vi "FaulhaberV3-Ascii_V1.vi"() -> (1 "searchnames":string[](array[string]), 2 "ID":u32[](array[numeric]), 3 "Faulhaber Objects":T3(array[cluster]))   [LabVIEW 2011] (continued)
"Default"="0", "Kommentart"=""}, {"ID"=621150254, "Name"="Encoder compensation_Value 45", "type"=enum."S16", "rw"=enum."rw", "lowLimit"="-32768", "highLimit"="32767", "Default"="0", "Kommentart"=""}, {"ID"=621150255, "Name"="Encoder compensation_Value 46", "type"=enum."S16", "rw"=enum."rw", "lowLimit"="-32768", "highLimit"="32767", "Default"="0", "Kommentart"=""}, {"ID"=621150256, "Name"="Encoder compensation_Value 47", "type"=enum."S16", "rw"=enum."rw", "lowLimit"="-32768", "highLimit"="32767", "Default"="0", "Kommentart"=""}, {"ID"=621150257, "Name"="Encoder compensation_Value 48", "type"=enum."S16", "rw"=enum."rw", "lowLimit"="-32768", "highLimit"="32767", "Default"="0", "Kommentart"=""}, {"ID"=621150258, "Name"="Encoder compensation_Value 49", "type"=enum."S16", "rw"=enum."rw", "lowLimit"="-32768", "highLimit"="32767", "Default"="0", "Kommentart"=""}, {"ID"=621150259, "Name"="Encoder compensation_Value 50", "type"=enum."S16", "rw"=enum."rw", "lowLimit"="-32768", "highLimit"="32767", "Default"="0", "Kommentart"=""}, {"ID"=621150260, "Name"="Encoder compensation_Value 51", "type"=enum."S16", "rw"=enum."rw", "lowLimit"="-32768", "highLimit"="32767", "Default"="0", "Kommentart"=""}, {"ID"=621150261, "Name"="Encoder compensation_Value 52", "type"=enum."S16", "rw"=enum."rw", "lowLimit"="-32768", "highLimit"="32767", "Default"="0", "Kommentart"=""}, {"ID"=621150262, "Name"="Encoder compensation_Value 53", "type"=enum."S16", "rw"=enum."rw", "lowLimit"="-32768", "highLimit"="32767", "Default"="0", "Kommentart"=""}, {"ID"=621150263, "Name"="Encoder compensation_Value 54", "type"=enum."S16", "rw"=enum."rw", "lowLimit"="-32768", "highLimit"="32767", "Default"="0", "Kommentart"=""}, {"ID"=621150264, "Name"="Encoder compensation_Value 55", "type"=enum."S16", "rw"=enum."rw", "lowLimit"="-32768", "highLimit"="32767", "Default"="0", "Kommentart"=""}, {"ID"=621150265, "Name"="Encoder compensation_Value 56", "type"=enum."S16", "rw"=enum."rw", "lowLimit"="-32768", "highLimit"="32767", "Default"="0", "Kommentart"=""}, {"ID"=621150266, "Name"="Encoder compensation_Value 57", "type"=enum."S16", "rw"=enum."rw", "lowLimit"="-32768", "highLimit"="32767", "Default"="0", "Kommentart"=""}, {"ID"=621150267, "Name"="Encoder compensation_Value 58", "type"=enum."S16", "rw"=enum."rw", "lowLimit"="-32768", "highLimit"="32767", "Default"="0", "Kommentart"=""}, {"ID"=621150268, "Name"="Encoder compensation_Value 59", "type"=enum."S16", "rw"=enum."rw", "lowLimit"="-32768", "highLimit"="32767", "Default"="0", "Kommentart"=""}, {"ID"=621150269, "Name"="Encoder compensation_Value 60", "type"=enum."S16", "rw"=enum."rw", "lowLimit"="-32768", "highLimit"="32767", "Default"="0", "Kommentart"=""}, {"ID"=621150270, "Name"="Encoder compensation_Value 61", "type"=enum."S16", "rw"=enum."rw", "lowLimit"="-32768", "highLimit"="32767", "Default"="0", "Kommentart"=""}, {"ID"=621150271, "Name"="Encoder compensation_Value 62", "type"=enum."S16", "rw"=enum."rw", "lowLimit"="-32768", "highLimit"="32767", "Default"="0", "Kommentart"=""}, {"ID"=621150272, "Name"="Encoder compensation_Value 63", "type"=enum."S16", "rw"=enum."rw", "lowLimit"="-32768", "highLimit"="32767", "Default"="0", "Kommentart"=""}, {"ID"=621412352, "Name"="Pwm frequency", "type"=enum."U8", "rw"=enum."rw", "lowLimit"="1", "highLimit"="10", "Default"="4", "Kommentart"=""}, {"ID"=621740032, "Name"="250F_00", "type"=enum."U8", "rw"=enum."wo", "lowLimit"="0", "highLimit"="255", "Default"="0", "Kommentart"=""}, {"ID"=637534208, "Name"="Drive system gear_Number of entries", "type"=enum."U8", "rw"=enum."ro", "lowLimit"="", "highLimit"="", "Default"="2", "Kommentart"=""}, {"ID"=637534209, "Name"="Drive system gear_Gear ratio num", "type"=enum."U32", "rw"=enum."rw", "lowLimit"="1", "highLimit"="4294967295", "Default"="1", "Kommentart"=""}, {"ID"=637534210, "Name"="Drive system gear_Gear ratio den", "type"=enum."U32", "rw"=enum."rw", "lowLimit"="1", "highLimit"="4294967295", "Default"="1", "Kommentart"=""}, {"ID"=637599744, "Name"="Drive system load transmission_Number of entries", "type"=enum."U8", "rw"=enum."ro", "lowLimit"="", "highLimit"="", "Default"="3", "Kommentart"=""}, {"ID"=637599745, "Name"="Drive system load transmission_Load transmission", "type"=enum."U8", "rw"=enum."rw", "lowLimit"="0", "highLimit"="255", "Default"="", "Kommentart"=""}, {"ID"=637599746, "Name"="Drive system load transmission_Load transmission ratio num", "type"=enum."U32", "rw"=enum."rw", "lowLimit"="1", "highLimit"="4294967295", "Default"="1", "Kommentart"=""}, {"ID"=637599747, "Name"="Drive system load transmission_Load transmission ratio den", "type"=enum."U32", "rw"=enum."rw", "lowLimit"="1", "highLimit"="4294967295", "Default"="1", "Kommentart"=""}, {"ID"=637665280, "Name"="Drive system numbers_Number of entries", "type"=enum."U8", "rw"=enum."ro", "lowLimit"="", "highLimit"="", "Default"="3", "Kommentart"=""}, {"ID"=637665281, "Name"="Drive system numbers_Gear catalog number", "type"=enum."string", "rw"=enum."rw", "lowLimit"="", "highLimit"="", "Default"="0", "Kommentart"=""}, {"ID"=637665282, "Name"="Drive system numbers_Encoder cataloge number", "type"=enum."string", "rw"=enum."rw", "lowLimit"="", "highLimit"="", "Default"="0", "Kommentart"=""}, {"ID"=637665283, "Name"="Drive system numbers_Drive combination number", "type"=enum."string", "rw"=enum."rw", "lowLimit"="", "highLimit"="", "Default"="0", "Kommentart"=""}, {"ID"=637730816, "Name"="Drive system units_Number of entries", "type"=enum."U8", "rw"=enum."ro", "lowLimit"="", "highLimit"="", "Default"="2", "Kommentart"=""}, {"ID"=637730817, "Name"="Drive system units_Unit reference", "type"=enum."U8", "rw"=enum."rw", "lowLimit"="0", "highLimit"="255", "Default"="0", "Kommentart"=""}, {"ID"=637730818, "Name"="Drive system units_Unit names", "type"=enum."string", "rw"=enum."rw", "lowLimit"="", "highLimit"="", "Default"="0", "Kommentart"=""}, {"ID"=637796352, "Name"="Nominal voltage", "type"=enum."U16", "rw"=enum."rw", "lowLimit"="0", "highLimit"="65535", "Default"="", "Kommentart"=""}, {"ID"=637861888, "Name"="Drive system settings", "type"=enum."U32", "rw"=enum."rw", "lowLimit"="0", "highLimit"="4294967295", "Default"="", "Kommentart"=""}, {"ID"=638582784, "Name"="OEM DeviceData_Number of entries", "type"=enum."U8", "rw"=enum."ro", "lowLimit"="", "highLimit"="", "Default"="3", "Kommentart"=""}, {"ID"=638582785, "Name"="OEM DeviceData_OEM product descriptor ", "type"=enum."string", "rw"=enum."rw", "lowLimit"="", "highLimit"="", "Default"="0", "Kommentart"=""}, {"ID"=638582786, "Name"="OEM DeviceData_OEM product code", "type"=enum."string", "rw"=enum."rw", "lowLimit"="", "highLimit"="", "Default"="0", "Kommentart"=""}, {"ID"=638582787, "Name"="OEM DeviceData_OEM serial number", "type"=enum."U32", "rw"=enum."rw", "lowLimit"="0", "highLimit"="4294967295", "Default"="0", "Kommentart"=""}, {"ID"=805306368, "Name"="User programs_Number of entries", "type"=enum."U8", "rw"=enum."ro", "lowLimit"="", "highLimit"="", "Default"="8", "Kommentart"=""}, {"ID"=805306369, "Name"="User programs_User program 1 start address", "type"=enum."U16", "rw"=enum."rw", "lowLimit"="0", "highLimit"="65535", "Default"="0xFFFF", "Kommentart"=""}, {"ID"=805306370, "Name"="User programs_User program 2 start address", "type"=enum."U16", "rw"=enum."rw", "lowLimit"="0", "highLimit"="65535", "Default"="0xFFFF", "Kommentart"=""}, {"ID"=805306371, "Name"="User programs_User program 3 start address", "type"=enum."U16", "rw"=enum."rw", "lowLimit"="0", "highLimit"="65535", "Default"="0xFFFF", "Kommentart"=""}, {"ID"=805306372, "Name"="User programs_User program 4 start address", "type"=enum."U16", "rw"=enum."rw", "lowLimit"="0", "highLimit"="65535", "Default"="0xFFFF", "Kommentart"=""}, {"ID"=805306373, "Name"="User programs_User program 5 start address", "type"=enum."U16", "rw"=enum."rw", "lowLimit"="0", "highLimit"="65535", "Default"="0xFFFF", "Kommentart"=""}, {"ID"=805306374, "Name"="User programs_User program 6 start address", "type"=enum."U16", "rw"=enum."rw", "lowLimit"="0", "highLimit"="65535", "Default"="0xFFFF", "Kommentart"=""}, {"ID"=805306375, "Name"="User programs_User program 7 start address", "type"=enum."U16", "rw"=enum."rw", "lowLimit"="0", "highLimit"="65535", "Default"="0xFFFF", "Kommentart"=""}, {"ID"=805306376, "Name"="User programs_User program 8 start address", "type"=enum."U16", "rw"=enum."rw", "lowLimit"="0", "highLimit"="65535", "Default"="0xFFFF", "Kommentart"=""}, {"ID"=805371904, "Name"="Active program_Number of entries", "type"=enum."U8", "rw"=enum."ro", "lowLimit"="", "highLimit"="", "Default"="10", "Kommentart"=""}, {"ID"=805371905, "Name"="Active program_Actual program command", "type"=enum."U8", "rw"=enum."rw", "lowLimit"="0", "highLimit"="255", "Default"="0", "Kommentart"=""}, {"ID"=805371906, "Name"="Active program_Actual program number", "type"=enum."U8", "rw"=enum."rw", "lowLimit"="0", "highLimit"="255", "Default"="0", "Kommentart"=""}, {"ID"=805371907, "Name"="Active program_Actual program position", "type"=enum."U16", "rw"=enum."ro", "lowLimit"="", "highLimit"="", "Default"="", "Kommentart"=""}, {"ID"=805371908, "Name"="Active program_Actual program state", "type"=enum."U8", "rw"=enum."ro", "lowLimit"="", "highLimit"="", "Default"="", "Kommentart"=""}, {"ID"=805371909, "Name"="Active program_Breakpoint address", "type"=enum."U16", "rw"=enum."rw", "lowLimit"="0", "highLimit"="65535", "Default"="0xFFFF", "Kommentart"=""}, {"ID"=805371911, "Name"="Active program_Upload/Download buffer", "type"=enum."string", "rw"=enum."rw", "lowLimit"="", "highLimit"="", "Default"="0", "Kommentart"=""}, {"ID"=805371912, "Name"="Active program_Error state", "type"=enum."U8", "rw"=enum."ro", "lowLimit"="", "highLimit"="", "Default"="", "Kommentart"=""}, {"ID"=805371913, "Name"="Active program_Error code", "type"=enum."U16", "rw"=enum."ro", "lowLimit"="", "highLimit"="", "Default"="", "Kommentart"=""}, {"ID"=805371914, "Name"="Active program_Program memory", "type"=enum."U16", "rw"=enum."ro", "lowLimit"="", "highLimit"="", "Default"="0", "Kommentart"=""}, {"ID"=805437440, "Name"="Auto start program", "type"=enum."U8", "rw"=enum."rw", "lowLimit"="0", "highLimit"="8", "Default"="0", "Kommentart"=""}, {"ID"=805502976, "Name"="Access key", "type"=enum."U32", "rw"=enum."wo", "lowLimit"="0", "highLimit"="4294967295", "Default"="0", "Kommentart"=""}, {"ID"=805568512, "Name"="Debug user program_Number of entries", "type"=enum."U8", "rw"=enum."ro", "lowLimit"="", "highLimit"="", "Default"="2", "Kommentart"=""}, {"ID"=805568513, "Name"="Debug user program_Select variable", "type"=enum."U8", "rw"=enum."rw", "lowLimit"="0", "highLimit"="25", "Default"="0", "Kommentart"=""}, {"ID"=805568514, "Name"="Debug user program_Selected variable value", "type"=enum."S32", "rw"=enum."rw", "lowLimit"="-2147483648", "highLimit"="2147483647", "Default"="0", "Kommentart"=""}, {"ID"=805634048, "Name"="User program variables_Number of entries", "type"=enum."U8", "rw"=enum."ro", "lowLimit"="", "highLimit"="", "Default"="26", "Kommentart"=""}, {"ID"=805634049, "Name"="User program variables_User prog variable a", "type"=enum."S32", "rw"=enum."rw", "lowLimit"="-2147483648", "highLimit"="2147483647", "Default"="0", "Kommentart"=""}, {"ID"=805634050, "Name"="User program variables_User prog variable b", "type"=enum."S32", "rw"=enum."rw", "lowLimit"="-2147483648", "highLimit"="2147483647", "Default"="0", "Kommentart"=""}, {"ID"=805634051, "Name"="User program variables_User prog variable c", "type"=enum."S32", "rw"=enum."rw", "lowLimit"="-2147483648", "highLimit"="2147483647", "Default"="0", "Kommentart"=""}, {"ID"=805634052, "Name"="User program variables_User prog variable d", "type"=enum."S32", "rw"=enum."rw", "lowLimit"="-2147483648", "highLimit"="2147483647", "Default"="0", "Kommentart"=""}, {"ID"=805634053, "Name"="User program variables_User prog variable e", "type"=enum."S32", "rw"=enum."rw", "lowLimit"="-2147483648", "highLimit"="2147483647", "Default"="0", "Kommentart"=""}, {"ID"=805634054, "Name"="User program variables_User prog variable f", "type"=enum."S32", "rw"=enum."rw", "lowLimit"="-2147483648", "highLimit"="2147483647", "Default"="0", "Kommentart"=""}, {"ID"=805634055, "Name"="User program variables_User prog variable g", "type"=enum."S32", "rw"=enum."rw", "lowLimit"="-2147483648", "highLimit"="2147483647", "Default"="0", "Kommentart"=""}, {"ID"=805634056, "Name"="User program variables_User prog variable h", "type"=enum."S32", "rw"=enum."rw", "lowLimit"="-2147483648", "highLimit"="2147483647", "Default"="0", "Kommentart"=""}, {"ID"=805634057, "Name"="User program variables_User prog variable i", "type"=enum."S32", "rw"=enum."rw", "lowLimit"="-2147483648", "highLimit"="2147483647", "Default"="0", "Kommentart"=""}, {"ID"=805634058, "Name"="User program variables_User prog variable j", "type"=enum."S32", "rw"=enum."rw", "lowLimit"="-2147483648", "highLimit"="2147483647", "Default"="0", "Kommentart"=""}, {"ID"=805634059, "Name"="User program variables_User prog variable k", "type"=enum."S32", "rw"=enum."rw", "lowLimit"="-2147483648", "highLimit"="2147483647", "Default"="0", "Kommentart"=""}, {"ID"=805634060, "Name"="User program variables_User prog variable l", "type"=enum."S32", "rw"=enum."rw", "lowLimit"="-2147483648", "highLimit"="2147483647", "Default"="0", "Kommentart"=""}, {"ID"=805634061, "Name"="User program variables_User prog variable m", "type"=enum."S32", "rw"=enum."rw", "lowLimit"="-2147483648", "highLimit"="2147483647", "Default"="0", "Kommentart"=""}, {"ID"=805634062, "Name"="User program variables_User prog variable n", "type"=enum."S32", "rw"=enum."rw", "lowLimit"="-2147483648", "highLimit"="2147483647", "Default"="0", "Kommentart"=""}, {"ID"=805634063, "Name"="User program variables_User prog variable o", "type"=enum."S32", "rw"=enum."rw", "lowLimit"="-2147483648", "highLimit"="2147483647", "Default"="0", "Kommentart"=""}, {"ID"=805634064, "Name"="User program variables_User prog variable p", "type"=enum."S32", "rw"=enum."rw", "lowLimit"="-2147483648", "highLimit"="2147483647", "Default"="0", "Kommentart"=""}, {"ID"=805634065, "Name"="User program variables_User prog variable q", "type"=enum."S32", "rw"=enum."rw", "lowLimit"="-2147483648", "highLimit"="2147483647", "Default"="0", "Kommentart"=""}, {"ID"=805634066, "Name"="User program variables_User prog variable r", "type"=enum."S32", "rw"=enum."rw", "lowLimit"="-2147483648", "highLimit"="2147483647", "Default"="0", "Kommentart"=""}, {"ID"=805634067, "Name"="User program variables_User prog variable s", "type"=enum."S32", "rw"=enum."rw", "lowLimit"="-2147483648", "highLimit"="2147483647", "Default"="0", "Kommentart"=""}, {"ID"=805634068, "Name"="User program variables_User prog variable t", "type"=enum."S32", "rw"=enum."rw", "lowLimit"="-2147483648", "highLimit"="2147483647", "Default"="0", "Kommentart"=""}, {"ID"=805634069, "Name"="User program variables_User prog variable u", "type"=enum."S32", "rw"=enum."rw", "lowLimit"="-2147483648", "highLimit"="2147483647", "Default"="0", "Kommentart"=""}, {"ID"=805634070, "Name"="User program variables_User prog variable v", "type"=enum."S32", "rw"=enum."rw", "lowLimit"="-2147483648", "highLimit"="2147483647", "Default"="0", "Kommentart"=""}, {"ID"=805634071, "Name"="User program variables_User prog variable w", "type"=enum."S32", "rw"=enum."rw", "lowLimit"="-2147483648", "highLimit"="2147483647", "Default"="0", "Kommentart"=""}, {"ID"=805634072, "Name"="User program variables_User prog variable x", "type"=enum."S32", "rw"=enum."rw", "lowLimit"="-2147483648", "highLimit"="2147483647", "Default"="0", "Kommentart"=""}, {"ID"=805634073, "Name"="User program variables_User prog variable y", "type"=enum."S32", "rw"=enum."rw", "lowLimit"="-2147483648", "highLimit"="2147483647", "Default"="0", "Kommentart"=""}, {"ID"=805634074, "Name"="User program variables_User prog variable z", "type"=enum."S32", "rw"=enum."rw", "lowLimit"="-2147483648", "highLimit"="2147483647", "Default"="0", "Kommentart"=""}, {"ID"=805699584, "Name"="Scripting stack / Number of levels_Number of levels", "type"=enum."U8", "rw"=enum."ro", "lowLimit"="", "highLimit"="", "Default"="15", "Kommentart"=""}, {"ID"=805699585, "Name"="Scripting stack / Number of levels_Call stack level 0", "type"=enum."U16", "rw"=enum."ro", "lowLimit"="", "highLimit"="", "Default"="0x0", "Kommentart"=""}, {"ID"=805699586, "Name"="Scripting stack / Number of levels_Call stack level 1", "type"=enum."U16", "rw"=enum."ro", "lowLimit"="", "highLimit"="", "Default"="0x0", "Kommentart"=""}, {"ID"=805699587, "Name"="Scripting stack / Number of levels_Call stack level 2", "type"=enum."U16", "rw"=enum."ro", "lowLimit"="", "highLimit"="", "Default"="0x0", "Kommentart"=""}, {"ID"=805699588, "Name"="Scripting stack / Number of levels_Call stack level 3", "type"=enum."U16", "rw"=enum."ro", "lowLimit"="", "highLimit"="", "Default"="0x0", "Kommentart"=""}, {"ID"=805699589, "Name"="Scripting stack / Number of levels_Call stack level 4", "type"=enum."U16", "rw"=enum."ro", "lowLimit"="", "highLimit"="", "Default"="0x0", "Kommentart"=""}, {"ID"=805699590, "Name"="Scripting stack / Number of levels_Call stack level 5", "type"=enum."U16", "rw"=enum."ro", "lowLimit"="", "highLimit"="", "Default"="0x0", "Kommentart"=""}, {"ID"=805699591, "Name"="Scripting stack / Number of levels_Call stack level 6", "type"=enum."U16", "rw"=enum."ro", "lowLimit"="", "highLimit"="", "Default"="0x0", "Kommentart"=""}, {"ID"=805699592, "Name"="Scripting stack / Number of levels_Call stack level 7", "type"=enum."U16", "rw"=enum."ro", "lowLimit"="", "highLimit"="", "Default"="0x0", "Kommentart"=""}, {"ID"=805699593, "Name"="Scripting stack / Number of levels_Call stack level 8", "type"=enum."U16", "rw"=enum."ro", "lowLimit"="", "highLimit"="", "Default"="0x0", "Kommentart"=""}, {"ID"=805699594, "Name"="Scripting stack / Number of levels_Call stack level 9", "type"=enum."U16", "rw"=enum."ro", "lowLimit"="", "highLimit"="", "Default"="0x0", "Kommentart"=""}, {"ID"=805699595, "Name"="Scripting stack / Number of levels_Call stack level 10", "type"=enum."U16", "rw"=enum."ro", "lowLimit"="", "highLimit"="", "Default"="0x0", "Kommentart"=""}, {"ID"=805699596, "Name"="Scripting stack / Number of levels_Call stack level 11", "type"=enum."U16", "rw"=enum."ro", "lowLimit"="", "highLimit"="", "Default"="0x0", "Kommentart"=""}, {"ID"=805699597, "Name"="Scripting stack / Number of levels_Call stack level 12", "type"=enum."U16", "rw"=enum."ro", "lowLimit"="", "highLimit"="", "Default"="0x0", "Kommentart"=""}, {"ID"=805699598, "Name"="Scripting stack / Number of levels_Call stack level 13", "type"=enum."U16", "rw"=enum."ro", "lowLimit"="", "highLimit"="", "Default"="0x0", "Kommentart"=""}, {"ID"=805699599, "Name"="Scripting stack / Number of levels_Call stack level 14", "type"=enum."U16", "rw"=enum."ro", "lowLimit"="", "highLimit"="", "Default"="0x0", "Kommentart"=""}, {"ID"=806289408, "Name"="Variable access key", "type"=enum."U32", "rw"=enum."wo", "lowLimit"="0", "highLimit"="4294967295", "Default"="0", "Kommentart"=""}, {"ID"=806354944, "Name"="Program constants_Number of entries", "type"=enum."U8", "rw"=enum."ro", "lowLimit"="", "highLimit"="", "Default"="16", "Kommentart"=""}, {"ID"=806354945, "Name"="Program constants_Program constant 0", "type"=enum."S32", "rw"=enum."rw", "lowLimit"="-2147483648", "highLimit"="2147483647", "Default"="0", "Kommentart"=""}, {"ID"=806354946, "Name"="Program constants_Program constant 1", "type"=enum."S32", "rw"=enum."rw", "lowLimit"="-2147483648", "highLimit"="2147483647", "Default"="0", "Kommentart"=""}, {"ID"=806354947, "Name"="Program constants_Program constant 2", "type"=enum."S32", "rw"=enum."rw", "lowLimit"="-2147483648", "highLimit"="2147483647", "Default"="0", "Kommentart"=""}, {"ID"=806354948, "Name"="Program constants_Program constant 3", "type"=enum."S32", "rw"=enum."rw", "lowLimit"="-2147483648", "highLimit"="2147483647", "Default"="0", "Kommentart"=""}, {"ID"=806354949, "Name"="Program constants_Program constant 4", "type"=enum."S32", "rw"=enum."rw", "lowLimit"="-2147483648", "highLimit"="2147483647", "Default"="0", "Kommentart"=""}, {"ID"=806354950, "Name"="Program constants_Program constant 5", "type"=enum."S32", "rw"=enum."rw", "lowLimit"="-2147483648", "highLimit"="2147483647", "Default"="0", "Kommentart"=""}, {"ID"=806354951, "Name"="Program constants_Program constant 6", "type"=enum."S32", "rw"=enum."rw", "lowLimit"="-2147483648", "highLimit"="2147483647", "Default"="0", "Kommentart"=""}, {"ID"=806354952, "Name"="Program constants_Program constant 7", "type"=enum."S32", "rw"=enum."rw", "lowLimit"="-2147483648", "highLimit"="2147483647", "Default"="0", "Kommentart"=""}, {"ID"=806354953, "Name"="Program constants_Program constant 8", "type"=enum."S32", "rw"=enum."rw", "lowLimit"="-2147483648", "highLimit"="2147483647", "Default"="0", "Kommentart"=""}, {"ID"=806354954, "Name"="Program constants_Program constant 9", "type"=enum."S32", "rw"=enum."rw", "lowLimit"="-2147483648", "highLimit"="2147483647", "Default"="0", "Kommentart"=""}, {"ID"=806354955, "Name"="Program constants_Program constant 10", "type"=enum."S32", "rw"=enum."rw", "lowLimit"="-2147483648", "highLimit"="2147483647", "Default"="0", "Kommentart"=""}, {"ID"=806354956, "Name"="Program constants_Program constant 11", "type"=enum."S32", "rw"=enum."rw", "lowLimit"="-2147483648", "highLimit"="2147483647", "Default"="0", "Kommentart"=""}, {"ID"=806354957, "Name"="Program constants_Program constant 12", "type"=enum."S32", "rw"=enum."rw", "lowLimit"="-2147483648", "highLimit"="2147483647", "Default"="0", "Kommentart"=""}, {"ID"=806354958, "Name"="Program constants_Program constant 13", "type"=enum."S32", "rw"=enum."rw", "lowLimit"="-2147483648", "highLimit"="2147483647", "Default"="0", "Kommentart"=""}, {"ID"=806354959, "Name"="Program constants_Program constant 14", "type"=enum."S32", "rw"=enum."rw", "lowLimit"="-2147483648", "highLimit"="2147483647", "Default"="0", "Kommentart"=""}, {"ID"=806354960, "Name"="Program constants_Program constant 15", "type"=enum."S32", "rw"=enum."rw", "lowLimit"="-2147483648", "highLimit"="2147483647", "Default"="0", "Kommentart"=""}, {"ID"=1611071488, "Name"="Abort connection option code", "type"=enum."S16", "rw"=enum."unknown", "lowLimit"="", "highLimit"="", "Default"="", "Kommentart"=""}, {"ID"=1614807040, "Name"="Controlword", "type"=enum."U16", "rw"=enum."rw", "lowLimit"="0", "highLimit"="65535", "Default"="0x0", "Kommentart"=""}, {"ID"=1614872576, "Name"="Statusword", "type"=enum."U16", "rw"=enum."ro", "lowLimit"="0x0", "highLimit"="", "Default"="", "Kommentart"=""}, {"ID"=1616510976, "Name"="Quick-Stop option code", "type"=enum."S16", "rw"=enum."unknown", "lowLimit"="", "highLimit"="", "Default"="", "Kommentart"=""}, {"ID"=1616576512, "Name"="Shutdown option code", "type"=enum."S16", "rw"=enum."unknown", "lowLimit"="", "highLimit"="", "Default"="", "Kommentart"=""}, {"ID"=1616642048, "Name"="Disable operation option code", "type"=enum."S16", "rw"=enum."unknown", "lowLimit"="", "highLimit"="", "Default"="", "Kommentart"=""}, {"ID"=1616707584, "Name"="Halt option code", "type"=enum."S16", "rw"=enum."unknown", "lowLimit"="", "highLimit"="", "Default"="", "Kommentart"=""}, {"ID"=1616773120, "Name"="Fault reaction option code", "type"=enum."S16", "rw"=enum."unknown", "lowLimit"="", "highLimit"="", "Default"="", "Kommentart"=""}, {"ID"=1616904192, "Name"="Modes of operation", "type"=enum."S8", "rw"=enum."unknown", "lowLimit"="", "highLimit"="", "Default"="", "Kommentart"=""}, {"ID"=1616969728, "Name"="Modes of operation display", "type"=enum."S8", "rw"=enum."ro", "lowLimit"="", "highLimit"="", "Default"="", "Kommentart"=""}, {"ID"=1617035264, "Name"="Position demand value", "type"=enum."S32", "rw"=enum."ro", "lowLimit"="", "highLimit"="", "Default"="", "Kommentart"=""}, {"ID"=1617100800, "Name"="Position actual internal value", "type"=enum."S32", "rw"=enum."ro", "lowLimit"="", "highLimit"="", "Default"="", "Kommentart"=""}, {"ID"=1617166336, "Name"="Position actual value", "type"=enum."S32", "rw"=enum."ro", "lowLimit"="", "highLimit"="", "Default"="", "Kommentart"=""}, {"ID"=1617231872, "Name"="Following error window", "type"=enum."U32", "rw"=enum."rw", "lowLimit"="0", "highLimit"="4294967295", "Default"="", "Kommentart"=""}, {"ID"=1617297408, "Name"="Following error time out", "type"=enum."U16", "rw"=enum."rw", "lowLimit"="1", "highLimit"="65535", "Default"="", "Kommentart"=""}, {"ID"=1617362944, "Name"="Position window", "type"=enum."U32", "rw"=enum."rw", "lowLimit"="0", "highLimit"="4294967295", "Default"="", "Kommentart"=""}, {"ID"=1617428480, "Name"="Position window time", "type"=enum."U16", "rw"=enum."rw", "lowLimit"="1", "highLimit"="65535", "Default"="", "Kommentart"=""}, {"ID"=1617625088, "Name"="Velocity demand value", "type"=enum."S32", "rw"=enum."ro", "lowLimit"="", "highLimit"="", "Default"="", "Kommentart"=""}, {"ID"=1617690624, "Name"="Velocity actual value", "type"=enum."S32", "rw"=enum."ro", "lowLimit"="", "highLimit"="", "Default"="", "Kommentart"=""}, {"ID"=1617756160, "Name"="Velocity window", "type"=enum."U16", "rw"=enum."rw", "lowLimit"="0", "highLimit"="65535", "Default"="", "Kommentart"=""}, {"ID"=1617821696, "Name"="Velocity window time", "type"=enum."U16", "rw"=enum."rw", "lowLimit"="1", "highLimit"="65535", "Default"="", "Kommentart"=""}, {"ID"=1617887232, "Name"="Velocity threshold", "type"=enum."U16", "rw"=enum."rw", "lowLimit"="0", "highLimit"="65535", "Default"="", "Kommentart"=""}, {"ID"=1617952768, "Name"="Velocity threshold time", "type"=enum."U16", "rw"=enum."rw", "lowLimit"="1", "highLimit"="65535", "Default"="", "Kommentart"=""}, {"ID"=1618018304, "Name"="Target torque", "type"=enum."S16", "rw"=enum."rw", "lowLimit"="-32768", "highLimit"="32767", "Default"="0", "Kommentart"=""}, {"ID"=1618083840, "Name"="Max torque", "type"=enum."U16", "rw"=enum."ro", "lowLimit"="", "highLimit"="", "Default"="", "Kommentart"=""}, {"ID"=1618214912, "Name"="Torque demand", "type"=enum."S16", "rw"=enum."ro", "lowLimit"="", "highLimit"="", "Default"="", "Kommentart"=""}, {"ID"=1618411520, "Name"="Torque actual value", "type"=enum."S16", "rw"=enum."ro", "lowLimit"="", "highLimit"="", "Default"="", "Kommentart"=""}, {"ID"=1618477056, "Name"="Current actual value", "type"=enum."S16", "rw"=enum."ro", "lowLimit"="", "highLimit"="", "Default"="", "Kommentart"=""}, {"ID"=1618608128, "Name"="Target position", "type"=enum."S32", "rw"=enum."rw", "lowLimit"="-2147483648", "highLimit"="2147483647", "Default"="0", "Kommentart"=""}, {"ID"=1618673664, "Name"="Position range limit_Number of entries", "type"=enum."U8", "rw"=enum."ro", "lowLimit"="", "highLimit"="", "Default"="2", "Kommentart"=""}, {"ID"=1618673665, "Name"="Position range limit_Min position range limit", "type"=enum."S32", "rw"=enum."rw", "lowLimit"="-2147483648", "highLimit"="2147483647", "Default"="-2147483648", "Kommentart"=""}, {"ID"=1618673666, "Name"="Position range limit_Max position range limit", "type"=enum."S32", "rw"=enum."rw", "lowLimit"="-2147483648", "highLimit"="2147483647", "Default"="2147483647", "Kommentart"=""}, {"ID"=1618739200, "Name"="Home offset", "type"=enum."S32", "rw"=enum."rw", "lowLimit"="-2147483648", "highLimit"="2147483647", "Default"="0", "Kommentart"=""}, {"ID"=1618804736, "Name"="Software position limit_Number of entries", "type"=enum."U8", "rw"=enum."ro", "lowLimit"="", "highLimit"="", "Default"="2", "Kommentart"=""}, {"ID"=1618804737, "Name"="Software position limit_Min position limit", "type"=enum."S32", "rw"=enum."rw", "lowLimit"="-2147483648", "highLimit"="2147483647", "Default"="-2147483648", "Kommentart"=""}, {"ID"=1618804738, "Name"="Software position limit_Max position limit", "type"=enum."S32", "rw"=enum."rw", "lowLimit"="-2147483648", "highLimit"="2147483647", "Default"="2147483647", "Kommentart"=""}, {"ID"=1618870272, "Name"="Polarity", "type"=enum."U8", "rw"=enum."unknown", "lowLimit"="", "highLimit"="", "Default"="", "Kommentart"=""}, {"ID"=1619001344, "Name"="Max motor speed ", "type"=enum."U32", "rw"=enum."rw", "lowLimit"="1", "highLimit"="4294967295", "Default"="32767", "Kommentart"=""}, {"ID"=1619066880, "Name"="Profile velocity", "type"=enum."U32", "rw"=enum."rw", "lowLimit"="1", "highLimit"="4294967295", "Default"="32767", "Kommentart"=""}, {"ID"=1619197952, "Name"="Profile acceleration", "type"=enum."U32", "rw"=enum."rw", "lowLimit"="1", "highLimit"="32767", "Default"="30000", "Kommentart"=""}, {"ID"=1619263488, "Name"="Profile deceleration", "type"=enum."U32", "rw"=enum."rw", "lowLimit"="1", "highLimit"="32767", "Default"="30000", "Kommentart"=""}, {"ID"=1619329024, "Name"="Quick stop deceleration", "type"=enum."U32", "rw"=enum."rw", "lowLimit"="10", "highLimit"="32767", "Default"="30000", "Kommentart"=""}, {"ID"=1619394560, "Name"="Motion profile type", "type"=enum."S16", "rw"=enum."unknown", "lowLimit"="", "highLimit"="", "Default"="", "Kommentart"=""}, {"ID"=1619984384, "Name"="Position encoder resolution_Number of entries", "type"=enum."U8", "rw"=enum."ro", "lowLimit"="", "highLimit"="", "Default"="2", "Kommentart"=""}, {"ID"=1619984385, "Name"="Position encoder resolution_Encoder increments", "type"=enum."U32", "rw"=enum."ro", "lowLimit"="", "highLimit"="", "Default"="", "Kommentart"=""}, {"ID"=1619984386, "Name"="Position encoder resolution_Motor revolutions", "type"=enum."U32", "rw"=enum."ro", "lowLimit"="", "highLimit"="", "Default"="", "Kommentart"=""}, {"ID"=1620049920, "Name"="Velocity encoder resolution_Number of entries", "type"=enum."U8", "rw"=enum."ro", "lowLimit"="", "highLimit"="", "Default"="2", "Kommentart"=""}, {"ID"=1620049921, "Name"="Velocity encoder resolution_Encoder increments", "type"=enum."U32", "rw"=enum."ro", "lowLimit"="", "highLimit"="", "Default"="", "Kommentart"=""}, {"ID"=1620049922, "Name"="Velocity encoder resolution_Motor revolutions", "type"=enum."U32", "rw"=enum."ro", "lowLimit"="", "highLimit"="", "Default"="", "Kommentart"=""}, {"ID"=1620115456, "Name"="Gear ratio_Number of entries", "type"=enum."U8", "rw"=enum."ro", "lowLimit"="", "highLimit"="", "Default"="2", "Kommentart"=""}, {"ID"=1620115457, "Name"="Gear ratio_Motor shaft revolutions", "type"=enum."U32", "rw"=enum."rw", "lowLimit"="1", "highLimit"="4294967295", "Default"="1", "Kommentart"=""}, {"ID"=1620115458, "Name"="Gear ratio_Driving shaft revolutions", "type"=enum."U32", "rw"=enum."rw", "lowLimit"="1", "highLimit"="4294967295", "Default"="1", "Kommentart"=""}, {"ID"=1620180992, "Name"="Feed constant_Number of entries", "type"=enum."U8", "rw"=enum."ro", "lowLimit"="", "highLimit"="", "Default"="2", "Kommentart"=""}, {"ID"=1620180993, "Name"="Feed constant_Feed", "type"=enum."U32", "rw"=enum."rw", "lowLimit"="1", "highLimit"="4294967295", "Default"="4096", "Kommentart"=""}, {"ID"=1620180994, "Name"="Feed constant_Shaft revolutions", "type"=enum."U32", "rw"=enum."rw", "lowLimit"="1", "highLimit"="4294967295", "Default"="1", "Kommentart"=""}, {"ID"=1620443136, "Name"="Velocity factor_Number of entries", "type"=enum."U8", "rw"=enum."ro", "lowLimit"="", "highLimit"="", "Default"="2", "Kommentart"=""}, {"ID"=1620443137, "Name"="Velocity factor_Numerator", "type"=enum."U32", "rw"=enum."rw", "lowLimit"="1", "highLimit"="4294967295", "Default"="1", "Kommentart"=""}, {"ID"=1620443138, "Name"="Velocity factor_Divisor", "type"=enum."U32", "rw"=enum."rw", "lowLimit"="1", "highLimit"="4294967295", "Default"="4096", "Kommentart"=""}, {"ID"=1620574208, "Name"="Homing method", "type"=enum."S8", "rw"=enum."rw", "lowLimit"="-4", "highLimit"="37", "Default"="0", "Kommentart"=""}, {"ID"=1620639744, "Name"="Homing speeds_Number of entries", "type"=enum."U8", "rw"=enum."ro", "lowLimit"="", "highLimit"="", "Default"="2", "Kommentart"=""}, {"ID"=1620639745, "Name"="Homing speeds_Switch seek velocity", "type"=enum."U32", "rw"=enum."rw", "lowLimit"="0", "highLimit"="4294967295", "Default"="400", "Kommentart"=""}, {"ID"=1620639746, "Name"="Homing speeds_Homing speed", "type"=enum."U32", "rw"=enum."rw", "lowLimit"="0", "highLimit"="4294967295", "Default"="400", "Kommentart"=""}, {"ID"=1620705280, "Name"="Homing acceleration", "type"=enum."U32", "rw"=enum."rw", "lowLimit"="0", "highLimit"="4294967295", "Default"="50", "Kommentart"=""}, {"ID"=1622147072, "Name"="Position offset", "type"=enum."S32", "rw"=enum."rw", "lowLimit"="-2147483648", "highLimit"="2147483647", "Default"="0", "Kommentart"=""}, {"ID"=1622212608, "Name"="Velocity offset", "type"=enum."S32", "rw"=enum."rw", "lowLimit"="-2147483648", "highLimit"="2147483647", "Default"="0", "Kommentart"=""}, {"ID"=1622278144, "Name"="Torque offset", "type"=enum."S16", "rw"=enum."rw", "lowLimit"="-32768", "highLimit"="32767", "Default"="0", "Kommentart"=""}, {"ID"=1622671360, "Name"="Touch probe function", "type"=enum."U16", "rw"=enum."rw", "lowLimit"="", "highLimit"="", "Default"="0", "Kommentart"=""}, {"ID"=1622736896, "Name"="Touch probe status", "type"=enum."U16", "rw"=enum."ro", "lowLimit"="", "highLimit"="", "Default"="0x0000", "Kommentart"=""}, {"ID"=1622802432, "Name"="Touch probe 1 positive edge", "type"=enum."S32", "rw"=enum."ro", "lowLimit"="", "highLimit"="", "Default"="0x0000", "Kommentart"=""}, {"ID"=1622867968, "Name"="Touch probe 1 negative edge", "type"=enum."S32", "rw"=enum."ro", "lowLimit"="", "highLimit"="", "Default"="", "Kommentart"=""}, {"ID"=1622933504, "Name"="Touch probe 2 positive edge", "type"=enum."S32", "rw"=enum."ro", "lowLimit"="", "highLimit"="", "Default"="", "Kommentart"=""}, {"ID"=1622999040, "Name"="Touch probe 2 negative edge", "type"=enum."S32", "rw"=enum."ro", "lowLimit"="", "highLimit"="", "Default"="", "Kommentart"=""}, {"ID"=1623523328, "Name"="Max acceleration", "type"=enum."U32", "rw"=enum."rw", "lowLimit"="10", "highLimit"="32767", "Default"="30000", "Kommentart"=""}, {"ID"=1623588864, "Name"="Max deceleration", "type"=enum."U32", "rw"=enum."rw", "lowLimit"="10", "highLimit"="32767", "Default"="30000", "Kommentart"=""}, {"ID"=1624571904, "Name"="Touch probe 1 positive edge counter", "type"=enum."U16", "rw"=enum."ro", "lowLimit"="", "highLimit"="", "Default"="", "Kommentart"=""}, {"ID"=1624637440, "Name"="Touch probe 1 negative edge counter", "type"=enum."U16", "rw"=enum."ro", "lowLimit"="", "highLimit"="", "Default"="", "Kommentart"=""}, {"ID"=1624702976, "Name"="Touch probe 2 positive edge counter", "type"=enum."U16", "rw"=enum."ro", "lowLimit"="", "highLimit"="", "Default"="", "Kommentart"=""}, {"ID"=1624768512, "Name"="Touch probe 2 negative edge counter", "type"=enum."U16", "rw"=enum."ro", "lowLimit"="", "highLimit"="", "Default"="", "Kommentart"=""}, {"ID"=1625292800, "Name"="Positive torque limit value", "type"=enum."U16", "rw"=enum."rw", "lowLimit"="0", "highLimit"="6000", "Default"="2000", "Kommentart"=""}, {"ID"=1625358336, "Name"="Negative torque limit value", "type"=enum."U16", "rw"=enum."rw", "lowLimit"="0", "highLimit"="6000", "Default"="2000", "Kommentart"=""}, {"ID"=1626472448, "Name"="Position option code", "type"=enum."U16", "rw"=enum."unknown", "lowLimit"="", "highLimit"="", "Default"="", "Kommentart"=""}, {"ID"=1626603520, "Name"="Following error actual value", "type"=enum."S32", "rw"=enum."ro", "lowLimit"="", "highLimit"="", "Default"="", "Kommentart"=""}, {"ID"=1627193344, "Name"="Digital Inputs", "type"=enum."U32", "rw"=enum."ro", "lowLimit"="", "highLimit"="", "Default"="", "Kommentart"=""}, {"ID"=1627324416, "Name"="Target velocity", "type"=enum."S32", "rw"=enum."rw", "lowLimit"="-2147483648", "highLimit"="2147483647", "Default"="0", "Kommentart"=""}, {"ID"=1677918208, "Name"="Motor catalogue number", "type"=enum."string", "rw"=enum."ro", "lowLimit"="", "highLimit"="", "Default"="", "Kommentart"=""}, {"ID"=1694629888, "Name"="Supported drive modes", "type"=enum."U32", "rw"=enum."ro", "lowLimit"="", "highLimit"="", "Default"="", "Kommentart"=""}, {"ID"=1694695424, "Name"="Drive catalogue number", "type"=enum."string", "rw"=enum."const", "lowLimit"="", "highLimit"="", "Default"="0", "Kommentart"=""}] {"ID" format="%x"})   [LabVIEW 2011]
uses:
  Library/XML.llb/MSXML Element.ctl
  Library/XML.llb/MSXML attribute.ctl
  FaulaberType.ctl
  FaulhaberAccess.ctl
panel:
  out "size":i32
  out "size(s)":i32
  out "Array":T4[](array[typedef])
  out "CanObjects":string
